vi "Dequeue Byte.vi"(8 "error in":errorcluster, 11 "Buffer":refnum<data-value>) -> (0 "error out":errorcluster, 1 "buffer empty?":bool, 2 "byte":u8 format="%02x", 3 "Buffer":refnum<data-value>)   [LabVIEW 2013, in "CircularBuffer.lvlib" / "ByteFIFO.lvclass"]
doc: "This VI allows to input an array into the buffer. The location in the buffer is updated automatically.\n\nIf the input array is larger than the buffer then just take last elements of the input array and save them in the buffer. Also give a warning that this happened."
uses:
  ByteFIFO.lvclass
  VariantBuffer/VariantBuffer.lvclass
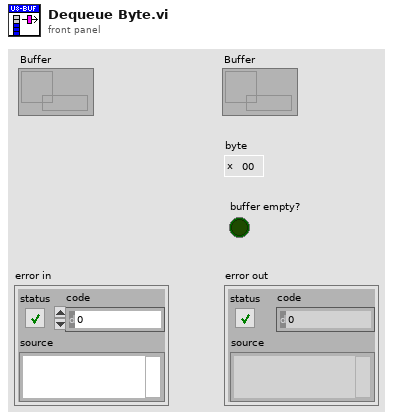
[diagram p1: front panel]
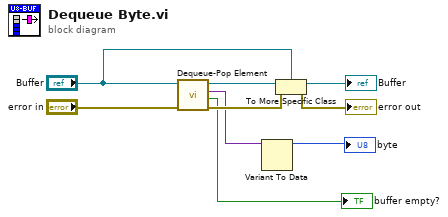
[diagram p0: block diagram]
diagram:
  n1 = call "Dequeue-Pop Element.vi"("error in"="error in", "Buffer in"="Buffer") -> ("error out"=w3:errorcluster, "buffer empty?"=→"buffer empty?":bool, "element"=w2:variant, "Buffer"=w5:refnum<data-value>)  [unwired: 6 in]
  n2 = Variant To Data(Variant=w2) -> (data=→"byte":u8)  [unwired: 2 in, 1 out]
  n3 = To More Specific Class(target class="Buffer", reference=w5, error in=w3) -> (specific class reference=→"Buffer":refnum<data-value>, error out=→"error out":errorcluster)
